vi "DAQNavi Read (Analog 1D U32 NChan NSamp).vi"(8 "error in (no error)":errorcluster, 9 "number of samples per channel to read":u32=1000, 10 "timeout":dbl=10.0 format="%0.2f", 11 "task in":i32) -> (0 "error out":errorcluster, 1 "markBuf":cluster{"Data Index":i64, "Src Id":i64}[](array[cluster]), 2 "data":u32[](array[numeric]), 3 "task out":i32)   [LabVIEW 2020]
uses:
  DAQNavi_LV.dll
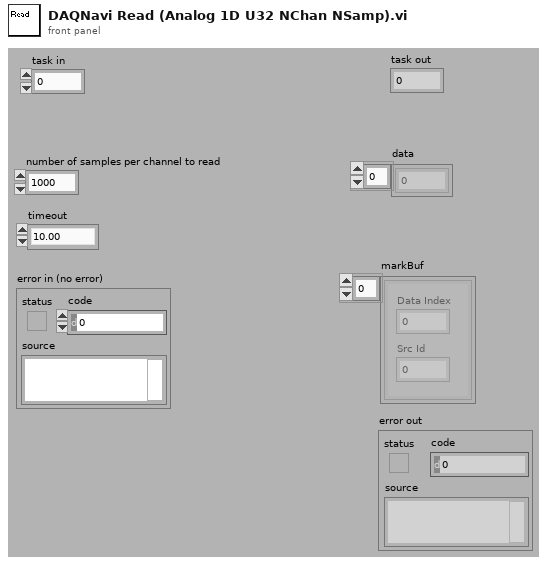
[diagram p1: front panel]
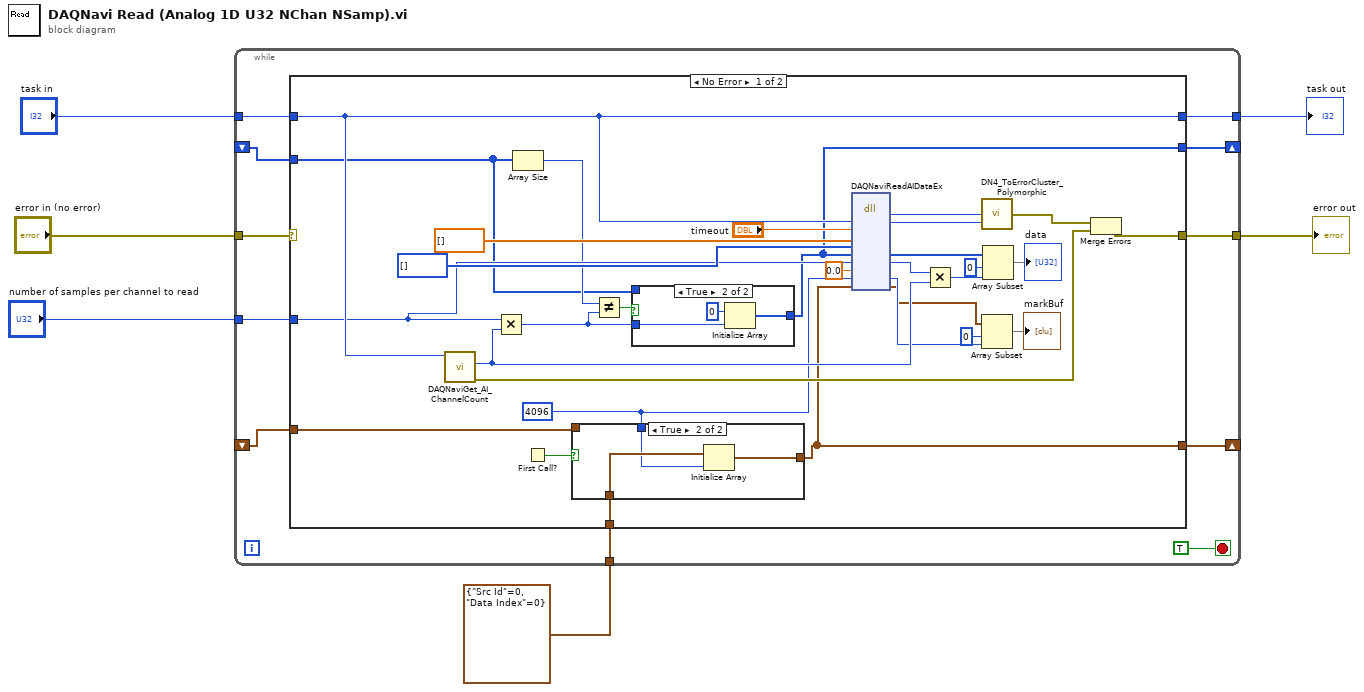
[diagram p0: block diagram]
diagram:
  n1 = while {
    tunnel: "task in" -> [w17]
    tunnel: "error in (no error)" -> [w16]
    tunnel: [w15] -> w4
    tunnel: [w14] -> w3
    tunnel: "number of samples per channel to read" -> [w13]
    shift-right: [w11] -> _
    shift-left: _ -> [w10]
    tunnel: cluster{"Src Id":i64, "Data Index":i64} {"Src Id"=0, "Data Index"=0} -> [w9]
    shift-right: [w8] -> _
    shift-left: _ -> [w7]
    stop <- TRUE stop-if-true
    n2 = case shown="No Error" w16 {
      selector: w16 -> [_ w59]
      tunnel: w17 -> [w41 w60]
      tunnel: [w41 w60] -> w15
      tunnel: [w39 w59] -> w14
      tunnel: w13 -> [w32 _]
      tunnel: [w29 w58] -> w11
      tunnel: w10 -> [w28 w58]
      tunnel: w9 -> [w26 _]
      tunnel: [w22 w57] -> w8
      tunnel: w7 -> [w25 w57]
      frame No Error {
        w23 = 4096
        n3 = call "DAQNaviGet_AI_ChannelCount.vi"("task in"=w41) -> ("error out"=w37:errorcluster, "channel count"=w35:i32)  [unwired: 1 in, 8 out]
        n4 = Multiply(x=w32, y=w35) -> (x*y=w40:u32)
        n5 = Array Size(array=w28) -> (size(s)=w30:i32)
        n6 = First Call?() -> (First Call?: T/F=w24:bool)
        n7 = case shown="True" w24 {
          tunnel: w26 -> [_ w52]
          tunnel: [w49 w51] -> w22
          tunnel: w25 -> [w49 _]
          tunnel: w23 -> [_ w50]
          frame False {
          }
          frame True {
            n8 = Initialize Array(w52, w50) -> (w51:cluster{"Src Id":i64, "Data Index":i64}[])
          }
        }
        n9 = Not Equal?(x=w30, y=w40) -> (x != y?=w31:bool)
        n10 = case shown="True" w31 {
          tunnel: w40 -> [_ w55]
          tunnel: [w53 w54] -> w29
          tunnel: w28 -> [w53 _]
          frame False {
          }
          frame True {
            n11 = Initialize Array(u32 0 ("element"), w55) -> (w54:u32[])
          }
        }
        n12 = dll-call lib="DAQNavi_LV.dll" fn="DAQNaviReadAIDataEx"("taskID"=w41, "timeout"="timeout", "scaledData"=dbl[] [], "rawData16"=u16[] [] ("rawData32"), "rawData32"=w29, "samples"=w32, "startTime"=0.0, "markCount"=w23, "markBuf"=w22) -> ("return type"=w46:i32, "taskID"=w33:i32, "rawData32"=w44:u32[], "samples"=w36:u32, "markCount"=w21:i32, "markBuf"=w19:cluster{"Src Id":i64, "Data Index":i64}[])  [unwired: 4 in, 5 out]
        n13 = Multiply(x=w36, y=w35) -> (x*y=w34:u32)
        n14 = call "DN4_ToErrorCluster_Polymorphic.vi"("task id"=w33, "error code"=w46) -> ("error out"=w38:errorcluster)  [unwired: 3 out]
        n15 = Array Subset(array=w19, index=0, length=w21) -> (→"markBuf":cluster{"Src Id":i64, "Data Index":i64}[])
        n16 = Array Subset(array=w44, index=0, length=w34) -> (→"data":u32[])
        n17 = Merge Errors(w38, w37) -> (w39:errorcluster)
      }
      frame Error {
      }
    }
  }
  "task out" <- w4
  "error out" <- w3
